vi "Temperature DAQ v1.1.vi"() -> ()   [LabVIEW 2013]
uses:
  <instrlib>/Lake Shore 336/Public/Data/Sensor Data (Single Reading).vi
  <instrlib>/Lake Shore 336/Lake Shore 336.lvlib
panel:
  in  "Heater Off":bool
  in  "Enter":bool
  in  "Setpoint":dbl format="%.5f"
  in  "Configure":bool
  in  "Output's Control Loop (1:1)":u16(ring)=1 items=["1"=1, "2"=2]
  in  "Input (0:None)":u16(ring)=1 items=["None", "A", "B", "C", "D"]
  in  "Mode":u16(ring)=1 items=["Off", "Closed Loop PID", "Zone", "Open Loop"]
  in  "Heater Out Display (1:Current)":u16(ring)=1 items=["Current"=1, "Power"=2]
  in  "Max Current (0:User Specified)":u16(ring) items=["User Specified", "0.707 A", "1.0 A", "1.141 A", "2.0 A"]
  in  "Heater Resistance (1:25 Ohms)":u16(ring)=1 items=["25 Ohms"=1, "50 Ohms"=2]
  in  "Max User Current (2.000)":dbl=2.0 format="%.3f"
  in  "Power Up Enable (F: Off)":bool
  in  "Gain (P)":dbl=50.0 format="%.1f"
  in  "Gain (I)":dbl=20.0 format="%.1f"
  in  "Gain (D)":dbl format="%.1f"
  in  "Manual Output (0.00 %)":dbl format="%.2f"
  in  "Range":u16(ring) items=["Off", "Low (On)", "Medium", "High"]
  in  "Input (0:A) 3":u16(ring)=3 items=["A", "B", "C", "D"]
  out "Sensor D: Radiation Shield":dbl
  in  "Input (0:A) 2":u16(ring)=2 items=["A", "B", "C", "D"]
  out "Sensor C: Top of the Magnet":dbl
  in  "Input (0:A) 1":u16(ring)=1 items=["A", "B", "C", "D"]
  out "Sensor B: 4k Plate":dbl
  in  "millisecond timer value":u32=100
  in  "stop":bool
  out "Sensor A: Sample Mount":dbl
  in  "Input (0:A) 0":u16(ring) items=["A", "B", "C", "D"]
  in  "Serial Configuration":T1={"Baud Rate"=57600, "Parity"=1, "Data Bits"=7, "Stop Bits"=10, "Flow Control"=0} {"Flow Control" items=["None", "XON/XOFF", "RTS/CTS", "XON/XOFF & RTS/CTS", "DTR/DSR", "XON/XOFF & DTR/DSR"]; "Stop Bits" items=["1.0"=10, "1.5"=15, "2.0"=20]; "Data Bits" items=["7"=7, "8"=8]; "Parity" items=["None", "Odd", "Even", "Mark", "Space"]; "Baud Rate" items=["300"=300, "600"=600, "1200"=1200, "2400"=2400, "4800"=4800, "9600"=9600, "19200"=19200, "38400"=38400, "57600"=57600]}
  in  "VISA resource name":refnum<visa-resource-name>="COM4"
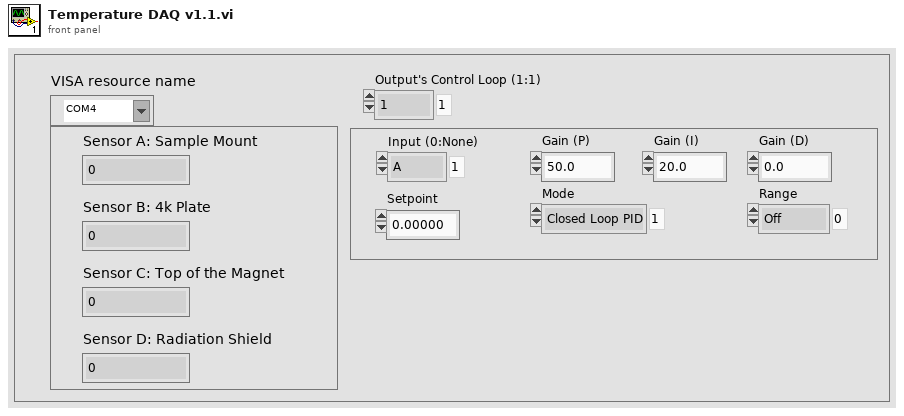
[diagram p1: front panel]
types:
  T1 = cluster{"Baud Rate":u32, "Parity":u16, "Data Bits":u16, "Stop Bits":u16, "Flow Control":u16}
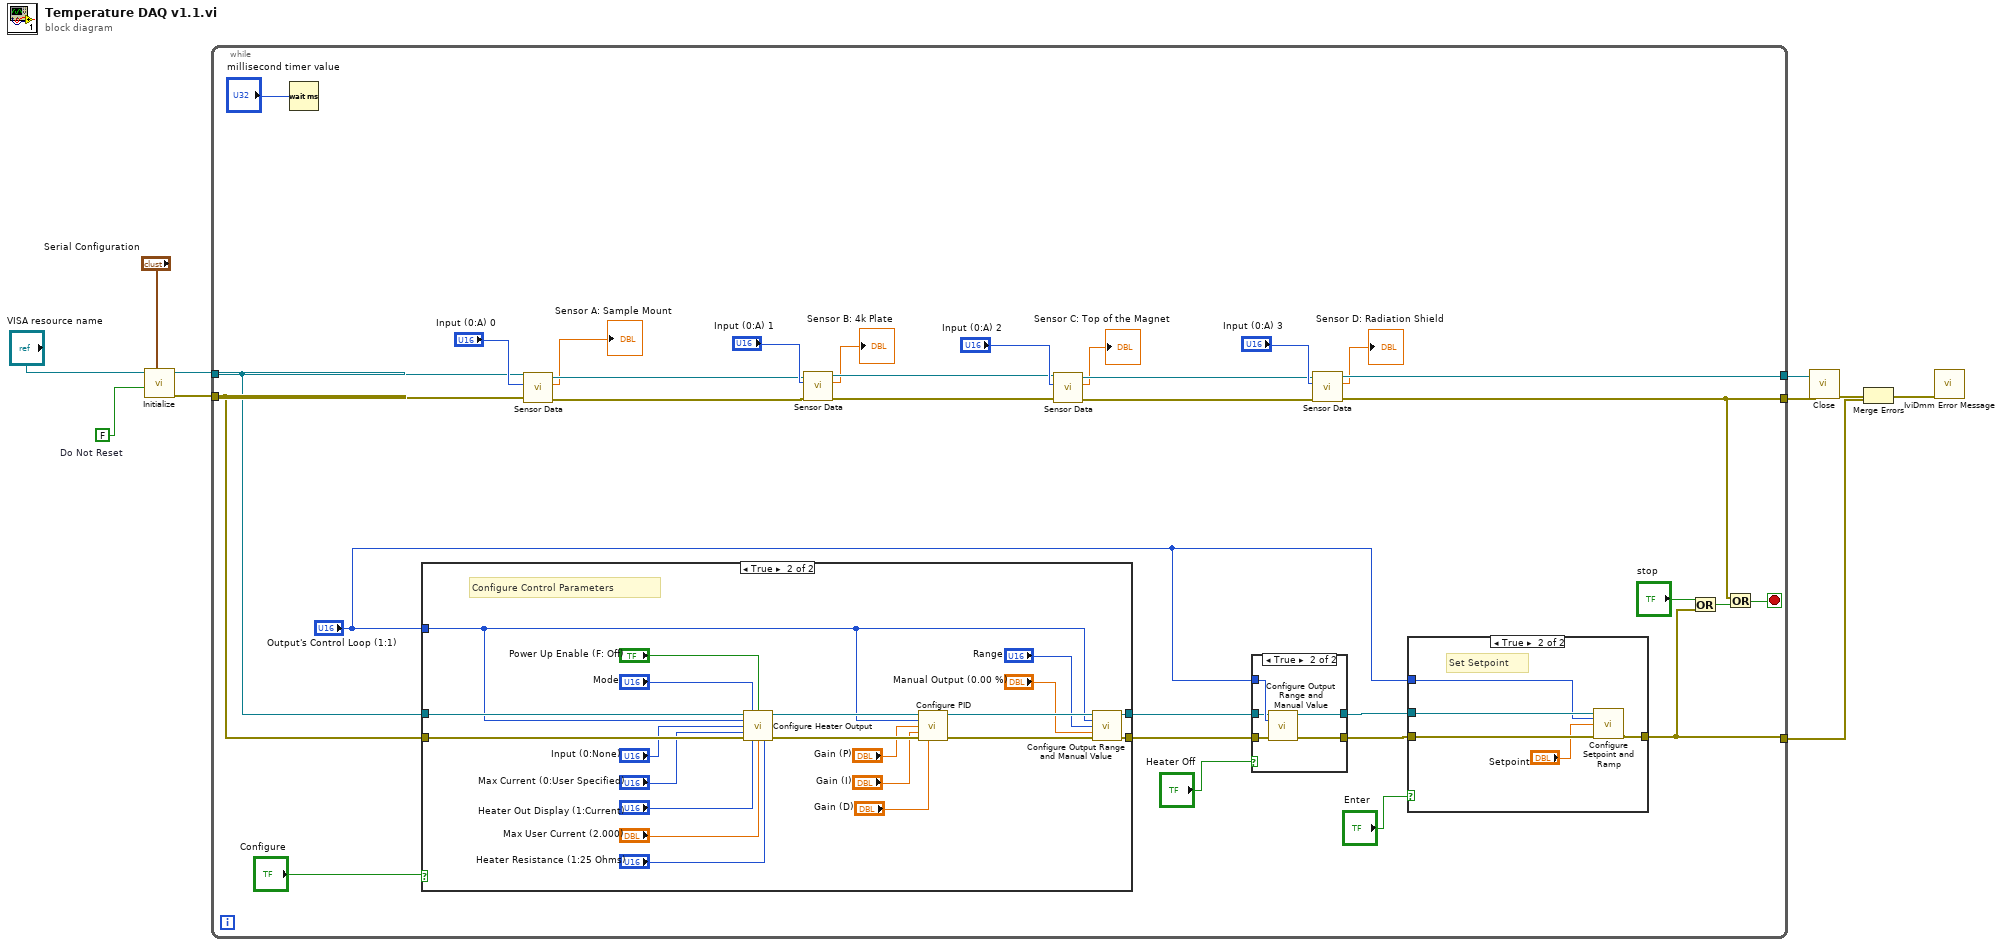
[diagram p0: block diagram]
diagram:
  w8 = FALSE  # Do Not Reset
  n1 = call <instrlib>:"Initialize.vi"("Serial Configuration"="Serial Configuration", "Reset (True)"=w8, "VISA resource name"="VISA resource name") -> ("error out"=w9:errorcluster, "VISA resource name out"=w10:refnum<visa-resource-name>)  [unwired: 7 in]
  n2 = while {
    tunnel: w10 -> [w23]
    tunnel: w9 -> [w22]
    tunnel: [w33] -> w5
    tunnel: [w24] -> w4
    tunnel: [w18] -> w2
    stop <- w29 stop-if-true
    n3 = Wait (ms)(milliseconds to wait="millisecond timer value") -> ()  [unwired: 1 out]
    n4 = case shown="True" "Configure" {
      tunnel: "Output's Control Loop (1:1)" -> [_ w63]
      tunnel: w23 -> [w56 w77]
      tunnel: w22 -> [w55 w76]
      tunnel: [w55 w71] -> w15
      tunnel: [w56 w57] -> w17
      frame False {
        # "Do Not Configure Control Parameters"
      }
      frame True {
        # "Configure Control Parameters"
        n5 = call <instrlib>:"Configure Heater Output.vi"("VISA resource name"=w77, "Mode (0:Off)"="Mode", "Power Up Enable (F: Off)"="Power Up Enable (F: Off)", "Heater Output (1:1)"=w63, "Input (0:None)"="Input (0:None)", "Max Current (0:User Specified)"="Max Current (0:User Specified)", "error in (no error)"=w76, "Heater Out Display (1:Current)"="Heater Out Display (1:Current)", "Max User Current (2.000)"="Max User Current (2.000)", "Heater Resistance (1:25 Ohms)"="Heater Resistance (1:25 Ohms)") -> ("VISA resource name out"=w74:refnum<visa-resource-name>, "error out"=w75:errorcluster)  [unwired: 4 in]
        n6 = call <instrlib>:"Configure PID.vi"("VISA resource name"=w74, "Output's Control Loop (1:1)"=w63, "Gain (P) (50.0)"="Gain (P)", "Reset (I) (20.0)"="Gain (I)", "error in (no error)"=w75, "Rate (D) (0.0 %)"="Gain (D)") -> ("VISA resource name out"=w73:refnum<visa-resource-name>, "error out"=w72:errorcluster)  [unwired: 8 in]
        n7 = call <instrlib>:"Configure Output Range and Manual Value.vi"("VISA resource name"=w73, "Output (1:1)"=w63, "Range (0:Off)"="Range", "Manual Output (0.00 %)"="Manual Output (0.00 %)", "error in (no error)"=w72) -> ("VISA resource name out"=w57:refnum<visa-resource-name>, "error out"=w71:errorcluster)  [unwired: 9 in]
      }
    }
    n8 = call-poly <instrlib>:"Sensor Data.vi"("error in (no error)"=w22, "Input (0:A)"="Input (0:A) 0", "VISA resource name"=w23) -> ("error out"=w32:errorcluster, "Sensor Data"=→"Sensor A: Sample Mount":dbl, "VISA resource name out"=w36:refnum<visa-resource-name>)  [unwired: 6 in]
    n9 = call-poly <instrlib>:"Sensor Data.vi"("error in (no error)"=w32, "Input (0:A)"="Input (0:A) 1", "VISA resource name"=w36) -> ("error out"=w31:errorcluster, "Sensor Data"=→"Sensor B: 4k Plate":dbl, "VISA resource name out"=w35:refnum<visa-resource-name>)  [unwired: 6 in]
    n10 = call-poly <instrlib>:"Sensor Data.vi"("error in (no error)"=w31, "Input (0:A)"="Input (0:A) 2", "VISA resource name"=w35) -> ("error out"=w30:errorcluster, "Sensor Data"=→"Sensor C: Top of the Magnet":dbl, "VISA resource name out"=w34:refnum<visa-resource-name>)  [unwired: 6 in]
    n11 = case shown="True" "Heater Off" {
      tunnel: "Output's Control Loop (1:1)" -> [_ w48]
      tunnel: w17 -> [w43 w47]
      tunnel: [w43 w46] -> w16
      tunnel: w15 -> [w42 w45]
      tunnel: [w42 w44] -> w14
      frame False {
      }
      frame True {
        n12 = call <instrlib>:"Configure Output Range and Manual Value.vi"("VISA resource name"=w47, "Output (1:1)"=w48, "error in (no error)"=w45) -> ("VISA resource name out"=w46:refnum<visa-resource-name>, "error out"=w44:errorcluster)  [unwired: 11 in]
      }
    }
    n13 = call-poly <instrlib>:"Sensor Data.vi"("error in (no error)"=w30, "Input (0:A)"="Input (0:A) 3", "VISA resource name"=w34) -> ("error out"=w24:errorcluster, "Sensor Data"=→"Sensor D: Radiation Shield":dbl, "VISA resource name out"=w33:refnum<visa-resource-name>)  [unwired: 6 in]
    n14 = case shown="True" "Enter" {
      tunnel: "Output's Control Loop (1:1)" -> [_ w52]
      tunnel: w16 -> [_ w53]
      tunnel: w14 -> [w49 w54]
      tunnel: [w49 w50] -> w18
      frame False {
        # "Do Not Set Setpoint"
      }
      frame True {
        # "Set Setpoint"
        n15 = call <instrlib>:"Configure Setpoint and Ramp.vi"("VISA resource name"=w53, "Output's Control Loop (1:1)"=w52, "Setpoint (0.00000)"="Setpoint", "error in (no error)"=w54) -> ("error out"=w50:errorcluster)  [unwired: 10 in, 1 out]
      }
    }
    n16 = Or(x="stop", y=w18) -> (x .or. y?=w20:bool)
    n17 = Or(x=w24, y=w20) -> (x .or. y?=w29:bool)
  }
  n18 = call <instrlib>:"Close.vi"("error in (no error)"=w4, "VISA resource name"=w5) -> ("error out"=w3:errorcluster)  [unwired: 9 in]
  n19 = Merge Errors(w3, w2) -> (w1:errorcluster)
  n20 = call <vilib>:"IviDmm Error Message.vi"("error in (no error)"=w1) -> ()  [unwired: 8 in, 3 out]
